vi "CreateFolderFromJSON.vi"() -> ()   [LabVIEW 2024]
uses:
  <userlib>/_OpenG.lib/file/file.llb/openg_file.lvlib
  <userlib>/_OpenG.lib/file/file.llb/Strip Path Extension - String__ogtk.vi
panel:
  out "error out":errorcluster
  in  "json file path":path
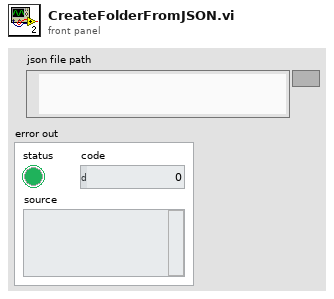
[diagram p1: front panel]
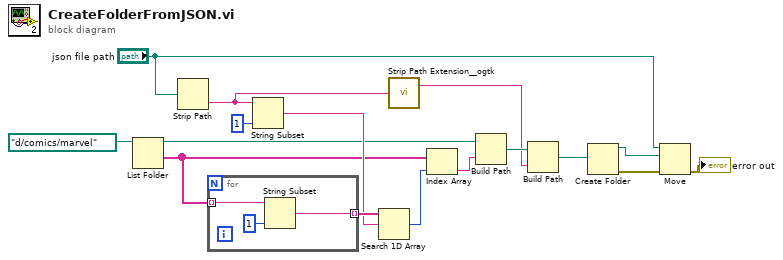
[diagram p0: block diagram]
diagram:
  n1 = List Folder(path=path "d:/comics/marvel") -> (path out=w9:path, folder names=w12:string[])  [unwired: 3 in, 2 out]
  n2 = Strip Path(path="json file path") -> (name=w2:string)  [unwired: 1 out]
  n3 = for {
    tunnel: w12 -> [w18] mode=indexing
    tunnel: [w17] -> w14 mode=indexing
    n4 = String Subset(string=w18, length (rest)=1 ("length (rest)")) -> (substring=w17:string)  [unwired: 1 in]
  }
  n5 = String Subset(string=w2, length (rest)=1 ("length (rest)")) -> (substring=w13:string)  [unwired: 1 in]
  n6 = Search 1D Array(1D array=w14, element=w13) -> (index of element=w11:i32)  [unwired: 1 in]
  n7 = call-poly <userlib>:"Strip Path Extension__ogtk.vi"("path"=w2) -> ("root"=w1:string)  [unwired: 1 out]
  n8 = Index Array(array=w12, index=w11) -> (element=w10:string)
  n9 = Build Path(base path=w9, name or relative path=w10) -> (appended path=w3:path)
  n10 = Build Path(base path=w3, name or relative path=w1) -> (appended path=w6:path)
  n11 = Create Folder(path (use dialog)=w6) -> (created path=w4:path, error out=w5:errorcluster)  [unwired: 2 in, 1 out]
  n12 = Move(source path="json file path", error in=w5, 10:w4) -> (error out=→"error out":errorcluster)  [unwired: 2 in, 2 out]
